vi "panel_update_status_string.vi"(8 "error in (no error)":errorcluster, 10 "String":string, 11 "lightfield_panel in":refnum<class "lightfield_panel.lvclass">) -> (0 "error out":errorcluster, 3 "lightfield_panel out":refnum<class "lightfield_panel.lvclass">)   [LabVIEW 2015, in "lightfield_panel.lvclass"]
uses:
  lightfield_panel.lvclass
  lightfield_panel.lvclass/lightfield_panel.ctl
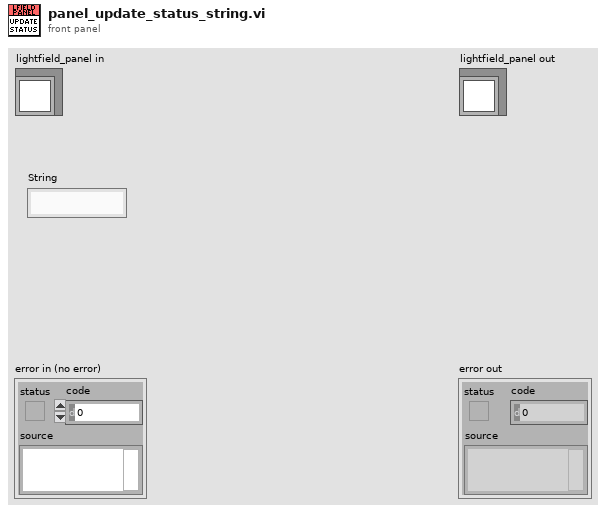
[diagram p1: front panel]
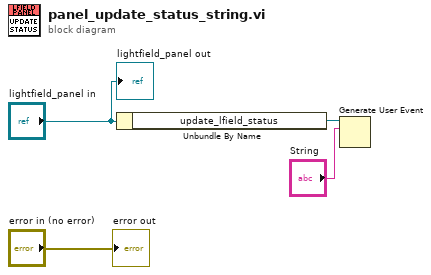
[diagram p0: block diagram]
diagram:
  n1 = Unbundle By Name("lightfield_panel in") -> ("update_lfield_status"=w4:refnum<user-event>)
  n2 = Generate User Event(user event=w4, event data cluster="String") -> ()  [unwired: 2 in, 2 out]
  "error out" <- "error in (no error)"
  "lightfield_panel out" <- "lightfield_panel in"
